vi "NumIntegrate_Rkdp_Func_A.vi"(9 "Col":i32, 11 "Row":i32) -> (3 "RKDP_A":dbl)   [LabVIEW 2019, in "Trajectory_Library.lvlib"]
doc: "Internal function used by Rkdp_Impl.vi\n\nInputs:\n - Row -- Row to look up ( 0 - 6 )\n - Column -- Column value to look up ( 0 - 6 )\n\nOutputs:\n - A -- Value looked up by index."
uses:
  Trajectory_Library.lvlib
  <vilib>/Analysis/Matrix/Datatypes/RealMatrix.ctl
  <vilib>/Analysis/Matrix/NI_Matrix.lvlib
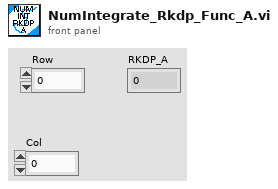
[diagram p1: front panel]
types:
  T1 = typedef "NI_Matrix.lvlib/RealMatrix.ctl" = dbl[][]
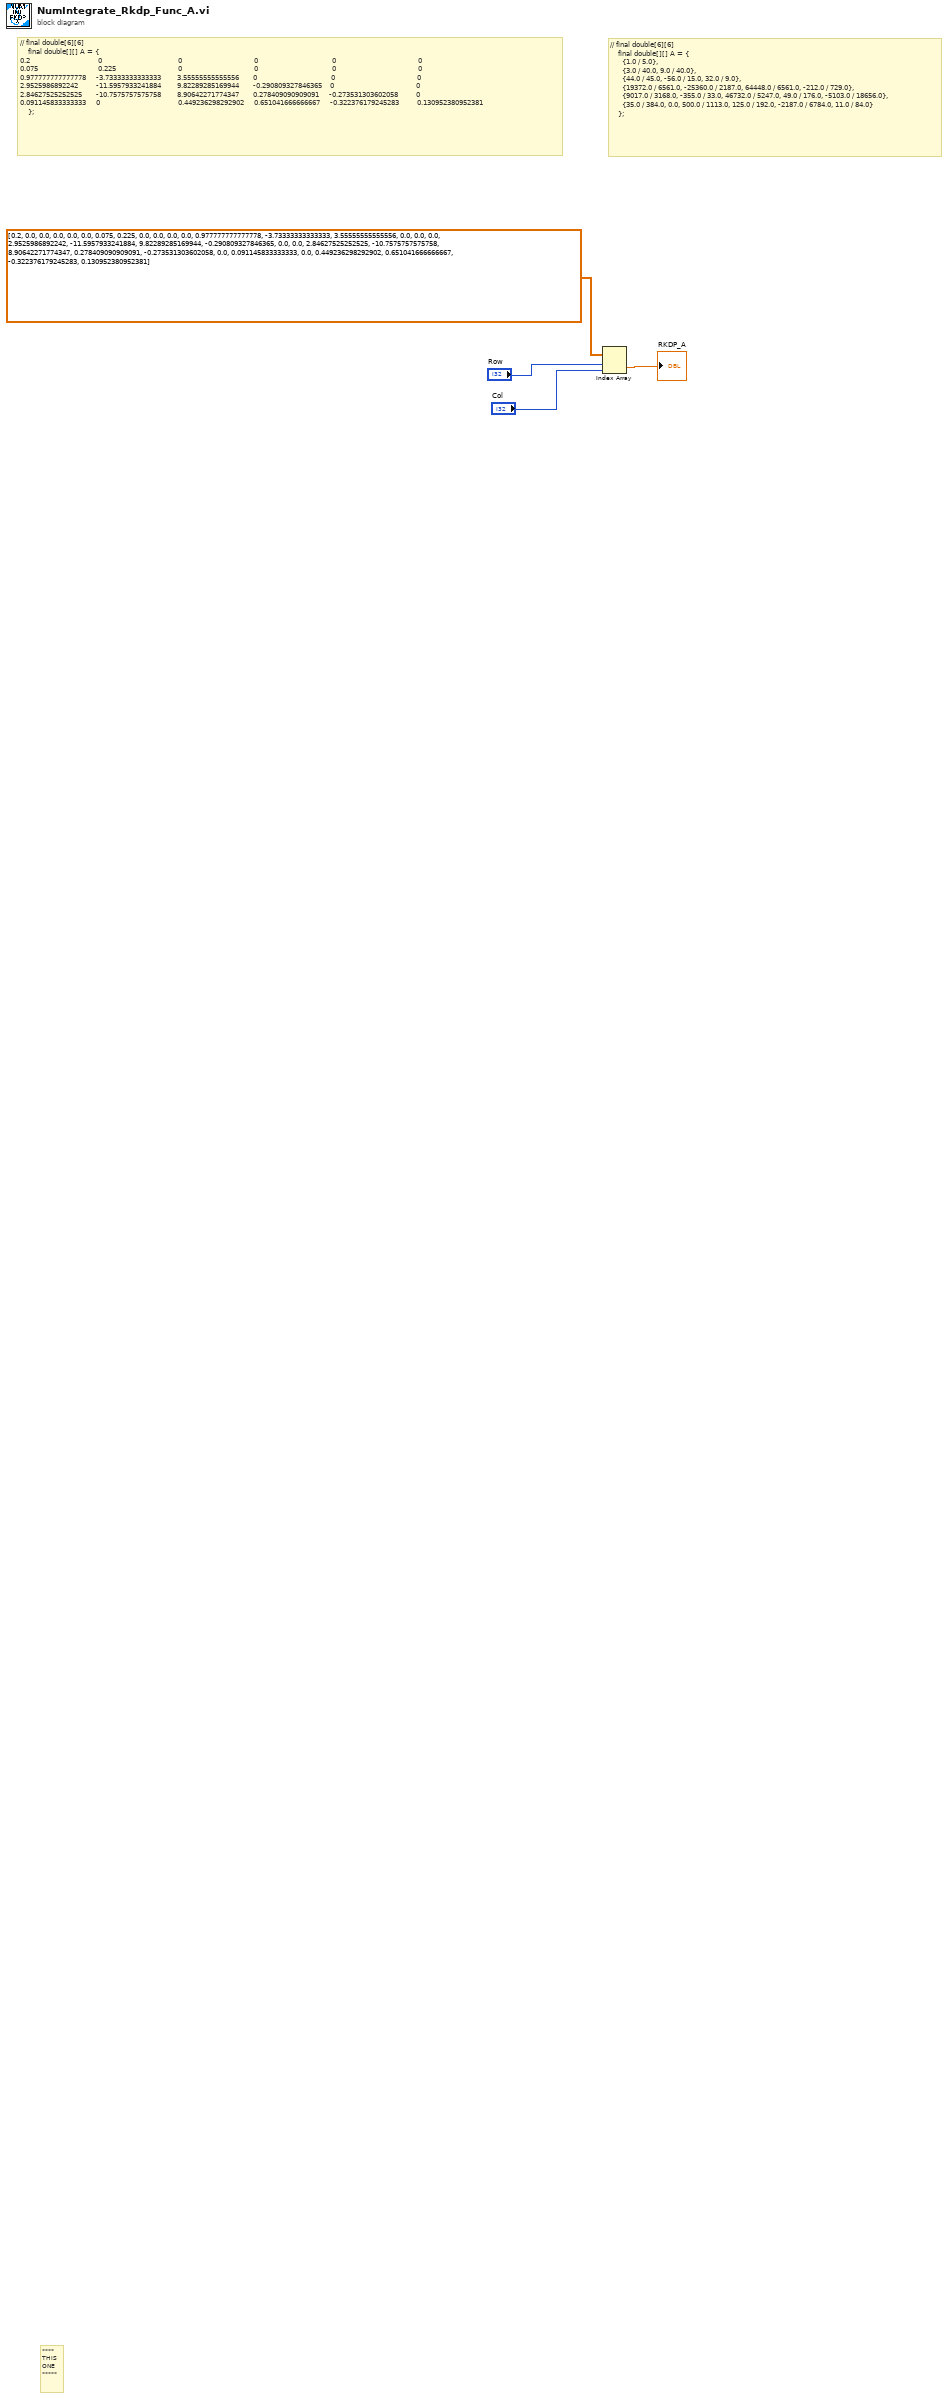
[diagram p0: block diagram]
diagram:
  # "// final double[6][6]\t\t\t\t\t\n    final double[][] A = {\t\t\t\t\t\n0.2\t                                 0\t                                     0\t                                   0  \t                                  0  \t                                      0\n0.075\t                             0.225\t                              0                               \t    0\t                                    0\t                                        0\n0.977777777777778  \t  -3.73333333333333\t       3.55555555555556\t      0\t                                    0\t                                        0\n2.9525986892242\t        -11.5957933241884\t       9.82289285169944\t      -0.290809327846365\t   0\t                                        0\n2.84627525252525\t      -10.7575757575758\t       8.90642271774347\t      0.278409090909091\t    -0.273531303602058\t        0\n0.091145833333333\t    0\t                                      0.449236298292902\t    0.651041666666667\t    -0.322376179245283\t        0.130952380952381\n    };"
  # "// final double[6][6]\n    final double[][] A = {\n      {1.0 / 5.0},\n      {3.0 / 40.0, 9.0 / 40.0},\n      {44.0 / 45.0, -56.0 / 15.0, 32.0 / 9.0},\n      {19372.0 / 6561.0, -25360.0 / 2187.0, 64448.0 / 6561.0, -212.0 / 729.0},\n      {9017.0 / 3168.0, -355.0 / 33.0, 46732.0 / 5247.0, 49.0 / 176.0, -5103.0 / 18656.0},\n      {35.0 / 384.0, 0.0, 500.0 / 1113.0, 125.0 / 192.0, -2187.0 / 6784.0, 11.0 / 84.0}\n    };"
  # "****\nTHIS\nONE\n*****"
  n1 = Index Array(array=T1 [[0.2, 0.0, 0.0, 0.0, 0.0, 0.0], [0.075, 0.225, 0.0, 0.0, 0.0, 0.0], [0.977777777777778, -3.73333333333333, 3.55555555555556, 0.0, 0.0, 0.0], [2.9525986892242, -11.5957933241884, 9.82289285169944, -0.290809327846365, 0.0, 0.0], [2.84627525252525, -10.7575757575758, 8.90642271774347, 0.278409090909091, -0.273531303602058, 0.0], [0.091145833333333, 0.0, 0.449236298292902, 0.651041666666667, -0.322376179245283, 0.130952380952381]] ("matrix"), index (row)="Row", index (col)="Col") -> (element=→"RKDP_A":dbl)
